vi "Test-server-message.vi"(8 "error in (no error)":errorcluster, 10 "Message":refnum<class "Message.lvclass">, 11 "ModComm in":T2) -> (0 "error out":errorcluster, 1 "Server message type":T1, 2 "Message dup":refnum<class "Message.lvclass">, 3 "ModComm out":T2, 4 "Server message?":bool)   [LabVIEW 2013, in "SLMServer.lvlib" / "SLMServer.lvclass"]
uses:
  SLMServer.lvclass
  Object-reference.ctl
  SA-SLMAPI/Sources/Message.lvclass
  Server-messages.ctl
  SA-SLMAPI/Sources/Message.lvclass/Message.ctl
  SA-SLMAPI/Sources/Read Message type.vi
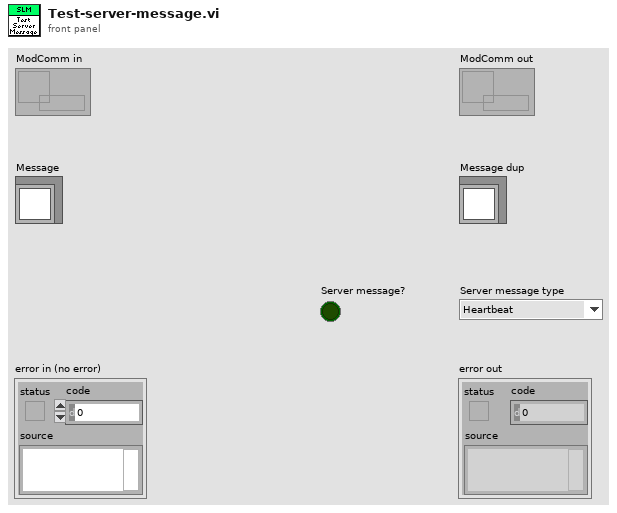
[diagram p1: front panel]
types:
  T1 = typedef "SLMServer.lvlib/SLMServer.lvclass/Server-messages.ctl" = enum16{"Heartbeat", "Error", "Start client", "Client stopped", "Get clients"}
  T2 = typedef "SLMServer.lvlib/SLMServer.lvclass/Object-reference.ctl" = refnum<data-value>
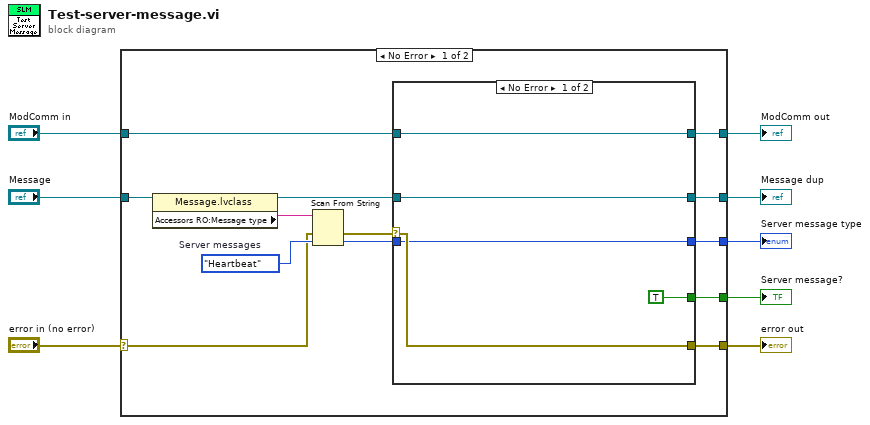
[diagram p0: block diagram]
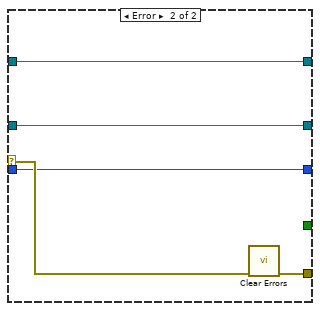
[diagram p2: hidden frame]
diagram:
  n1 = case shown="No Error" "error in (no error)" {
    selector: "error in (no error)" -> [w16 w34]
    tunnel: [w10 w34] -> w7
    tunnel: [w12 w33] -> w5
    tunnel: "ModComm in" -> [w19 w33]
    tunnel: "Message" -> [w21 w32]
    tunnel: [w11 w32] -> w3
    tunnel: [w13 _] -> w2
    tunnel: [w9 _] -> w1
    frame No Error {
      w17 = Server-messages."Heartbeat"  # Server messages
      n2 = property class="Message.lvclass"(reference=w21) -> (reference out=w18:refnum<class "Message.lvclass">, "Accessors RO:Message type"=w20:string)  [unwired: 1 in, 1 out]
      n3 = Scan From String(input string=w20, error in=w16, default 1=w17) -> (error out=w15:errorcluster, output 1=w14:T1)  [unwired: 2 in, 2 out]
      n4 = case shown="No Error" w15 {
        selector: w15 -> [w23 w28]
        tunnel: w19 -> [w24 w31]
        tunnel: w18 -> [w25 w30]
        tunnel: w14 -> [w22 w27]
        tunnel: [TRUE _] -> w13
        tunnel: [w24 w31] -> w12
        tunnel: [w25 w30] -> w11
        tunnel: [w23 w29] -> w10
        tunnel: [w22 w27] -> w9
        frame No Error {
        }
        frame Error {
          n5 = call <vilib>:"Clear Errors.vi"("error in (no error)"=w28) -> ("error out"=w29:errorcluster)  [unwired: 6 in]
        }
      }
    }
    frame Error {
    }
  }
  "error out" <- w7
  "ModComm out" <- w5
  "Message dup" <- w3
  "Server message?" <- w2
  "Server message type" <- w1
